vi "Visa_Write read_UI GETPIN.vi"(0 "NXP in":refnum<class "NXP.lvclass">, 1 "VISA resource name":refnum<visa-resource-name>, 2 "Command to Send":string, 3 "Expected Response":string, 4 "Buttons":bool[](array[boolean]), 5 "error in (no error)":errorcluster) -> (13 "Valor pin":bool, 14 "NXP out":refnum<class "NXP.lvclass">, 15 "VISA resource name":refnum<visa-resource-name>, 16 "Response":string, 17 "Port":string, 18 "PIN":string, 19 "error out":errorcluster)   [LabVIEW 2020, in "NXP.lvclass"]
uses:
  NXP.lvclass
  Abstract/Serial Device/Combo Box Devices.ctl
  Abstract/Serial Device/Combo Box Comandos.ctl
  UI Actor/UI Actor.lvclass
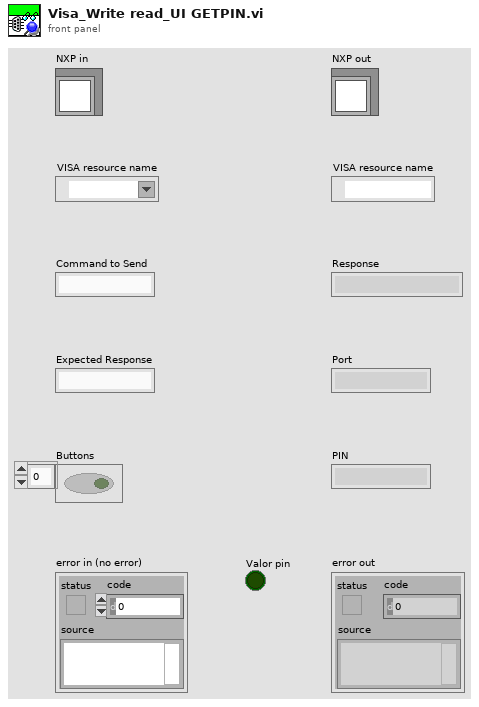
[diagram p1: front panel]
types:
  T1 = typedef "Combo Box Comandos.ctl" = string
  T2 = typedef "Combo Box Devices.ctl" = string
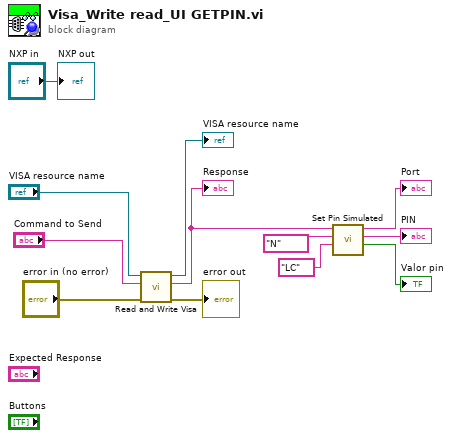
[diagram p0: block diagram]
diagram:
  n1 = call "Read and Write Visa.vi"("error in (no error)"="error in (no error)", "Command to Send"="Command to Send", "VISA Refnum in"="VISA resource name") -> ("error out"=→"error out":errorcluster, "Expected Response out"=w6:string, "VISA Refnum out"=→"VISA resource name":refnum<visa-resource-name>)  [unwired: 6 in]
  "Response" <- w6
  n2 = call "Set Pin Simulated.vi"("Command"=T1 "LC", "Serial Devide Brand"=T2 "N", "Command to Send"=w6) -> ("Pin"=→"Valor pin":bool, "Valor Pin"=→"PIN":string, "Puerto"=→"Port":string)  [unwired: 6 in]
  "NXP out" <- "NXP in"
